vi "XML.IntoVariant.vi"(8 "error in":errorcluster, 10 "XML file path":path=path "C:/Projects/TMOS-LINAK_TD4_ADV/Settings/HW_config.xml") -> (0 "error out":errorcluster, 1 "all parameter names":string[](array[string]), 2 "variant":variant)   [LabVIEW 2019, in "Tools.lvlib"]
uses:
  <vilib>/xml/Load XML File.vi
  <vilib>/xml/Close Reference(Node).vi
  Tools.lvlib
  <vilib>/xml/NI_XML.lvlib
panel:
  # "https://svn.tm-solutions.eu/svn/PL_0366_TMSPL_TMOS_Framework_Internal/branches/TMOS-LINAK_TD4_ADV/Procedures"
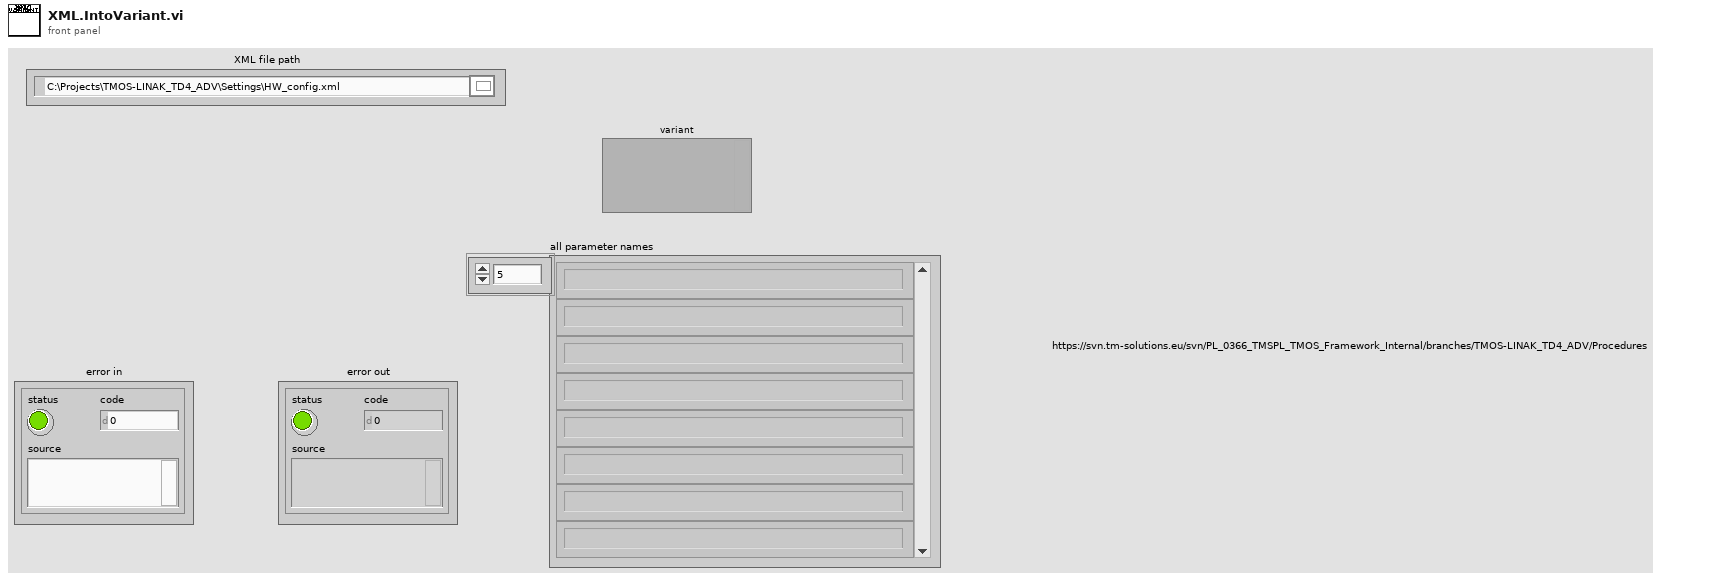
[diagram p1: front panel]
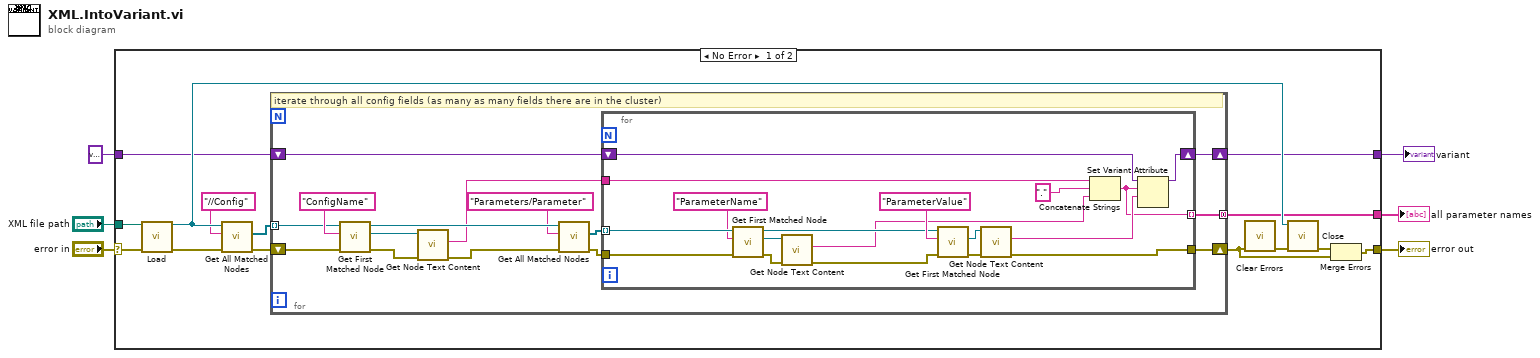
[diagram p0: block diagram]
diagram:
  n1 = case shown="No Error" "error in" {
    selector: "error in" -> [w19 w55]
    tunnel: [w17 w55] -> w6
    tunnel: "XML file path" -> [w20 _]
    tunnel: variant -> [w15 w54]
    tunnel: [w8 w54] -> w2
    tunnel: [w7 _] -> w1
    frame No Error {
      n2 = call-poly <vilib>:"Load.vi"("path to XML document"=w20, "error in (no error)"=w19) -> ("DOM document out"=w18:refnum<k20>, "error out"=w11:errorcluster)  [unwired: 11 in, 1 out]
      n3 = call <vilib>:"Get All Matched Nodes.vi"("error in (no error)"=w11, "XPath expression"="//Config", "node in"=w18) -> ("error out"=w14:errorcluster, "node result array"=w13:refnum<k20>[])  [unwired: 6 in, 1 out]
      n4 = for {
        tunnel: w13 -> [w22] mode=indexing
        shift-right: [w23] -> w10
        shift-left: w14 -> [w35]
        shift-right: [w24] -> w8
        shift-left: w15 -> [w26]
        tunnel: [w21] -> w7 mode=concatenating
        # "iterate through all config fields (as many as many fields there are in the cluster)"
        n5 = call <vilib>:"Get First Matched Node.vi"("error in (no error)"=w35, "XPath expression"="ConfigName", "node in"=w22) -> ("error out"=w32:errorcluster, "node result"=w33:refnum<k20>, "node out"=w31:refnum<k20>)  [unwired: 6 in]
        n6 = call <vilib>:"Get Node Text Content.vi"("error in (no error)"=w32, "node in"=w33) -> ("error out"=w28:errorcluster, "node text"=w25:string)  [unwired: 7 in, 1 out]
        n7 = call <vilib>:"Get All Matched Nodes.vi"("error in (no error)"=w28, "XPath expression"="Parameters/Parameter", "node in"=w31) -> ("error out"=w27:errorcluster, "node result array"=w29:refnum<k20>[])  [unwired: 6 in, 1 out]
        n8 = for {
          tunnel: w29 -> [w53] mode=indexing
          tunnel: w27 -> [w49]
          tunnel: w25 -> [w43]
          shift-right: [w39] -> w24
          shift-left: w26 -> [w48]
          tunnel: [w37] -> w23
          tunnel: [w36] -> w21 mode=indexing
          n9 = call <vilib>:"Get First Matched Node.vi"("error in (no error)"=w49, "XPath expression"="ParameterName", "node in"=w53) -> ("error out"=w46:errorcluster, "node result"=w47:refnum<k20>, "node out"=w50:refnum<k20>)  [unwired: 6 in]
          n10 = call <vilib>:"Get Node Text Content.vi"("error in (no error)"=w46, "node in"=w47) -> ("error out"=w45:errorcluster, "node text"=w42:string)  [unwired: 7 in, 1 out]
          n11 = call <vilib>:"Get First Matched Node.vi"("error in (no error)"=w45, "XPath expression"="ParameterValue", "node in"=w50) -> ("error out"=w44:errorcluster, "node result"=w38:refnum<k20>)  [unwired: 6 in, 1 out]
          n12 = call <vilib>:"Get Node Text Content.vi"("error in (no error)"=w44, "node in"=w38) -> ("error out"=w37:errorcluster, "node text"=w41:string)  [unwired: 7 in, 1 out]
          n13 = Concatenate Strings(w43, "." ("string"), w42) -> (w36:string)
          n14 = Set Variant Attribute(Variant=w48, name=w36, value=w41) -> (Variant out=w39:variant)  [unwired: 1 in, 2 out]
        }
      }
      n15 = call <vilib>:"Clear Errors.vi"("error in (no error)"=w10) -> ("error out"=w9:errorcluster)  [unwired: 5 in, 1 out]
      n16 = call-poly <vilib>:"Close.vi"("error in (no error)"=w9, "node"=w18) -> ("error out"=w16:errorcluster)  [unwired: 7 in]
      n17 = Merge Errors(w16, w10) -> (w17:errorcluster)
    }
    frame Error {
    }
  }
  "error out" <- w6
  "variant" <- w2
  "all parameter names" <- w1
